vi "flagspinner.vi"   [LabVIEW 2012, in "BlockParty4150.lvrbt"]
uses:
  BlockParty4150.lvrbt
  <vilib>/NXT/Block Support/NXT_ButtonSelector.ctl
  <vilib>/NXT/Hardware/Plugins/Tetrix DC Motor/TetrixDCMotorAddress.ctl
  <vilib>/NXT/NXTIO Xnodes/NXTIONodeSubVIs/TETRIX IO Move DC Motors.vi
  <vilib>/NXT/Subs/LVHSConnector.ctl
  <vilib>/NXT/NXTIO Xnodes/AddressXNode/NXTIOAddress.xnode
  <vilib>/NXT/NXTIO Xnodes/NXTIOXNode/NXTIO.xnode
  <vilib>/NXT/LegoClasses/BrickReference/BrickReference.lvclass
types:
  T1 = typedef "NXT_ButtonSelector.ctl" = u16
  T2 = typedef "TetrixDCMotorAddress.ctl" = i16
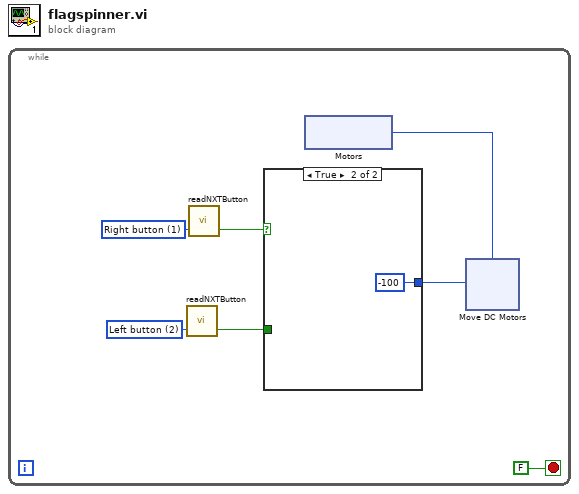
[diagram p0: block diagram]
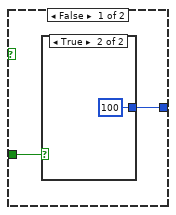
[diagram p2: hidden frame]
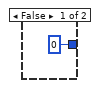
[diagram p3: hidden frame]
diagram:
  n1 = while {
    stop <- FALSE stop-if-true
    w5 = T1 1 items=["Enter button"=3, "Left button"=2, "Right button"=1] ("Button (Enter button)")
    w6 = T1 2 items=["Enter button"=3, "Left button"=2, "Right button"=1] ("Button (Enter button)")
    n2 = call <vilib>:"readNXTButton.vi"("Button (Enter button)"=w6) -> ("Yes/No"=w3:bool)  [unwired: 2 in, 1 out]
    n3 = call <vilib>:"readNXTButton.vi"("Button (Enter button)"=w5) -> ("Yes/No"=w4:bool)  [unwired: 2 in, 1 out]
    n4 = case shown="True" w4 {
      tunnel: w3 -> [w17 _]
      tunnel: [w16 i8 -100 ("Power/Speed 1")] -> w1
      frame False {
        n5 = case shown="True" w17 {
          tunnel: [i8 0 ("Power/Speed 1") i8 100 ("Power/Speed 1")] -> w16
          frame False {
          }
          frame True {
          }
        }
      }
      frame True {
      }
    }
    n6 = xnode "Motors"() -> ("Motor"=w2:T2)
    n7 = xnode "Move DC Motors"("Power/Speed 1"=w1, "Motors"=w2) -> ()  [unwired: 1 in, 1 out]
  }
